vi "W7X2DPut.vi"(0 "SigLabel":string, 1 "SigJSONbuffer":string, 3 "values":T1(array[cluster]), 4 "sample rate":u16, 5 "sample period":dbl, 6 "Unit":string, 7 "pulse_length":dbl, 8 "local storage only":bool, 17 "dimensions":i64[](array[numeric])=[1399090569999999999, -1]) -> (10 "headers parms":string, 12 "headers":string, 13 "Parlog error out":errorcluster, 14 "body":string, 15 "body Parlog":string, 18 "file path written":string)   [LabVIEW 2014]
uses:
  <vilib>/httpClient/POSTBuffer.vi
  <vilib>/httpClient/LabVIEWHTTPClient.lvlib
panel:
  out "JSON string":string
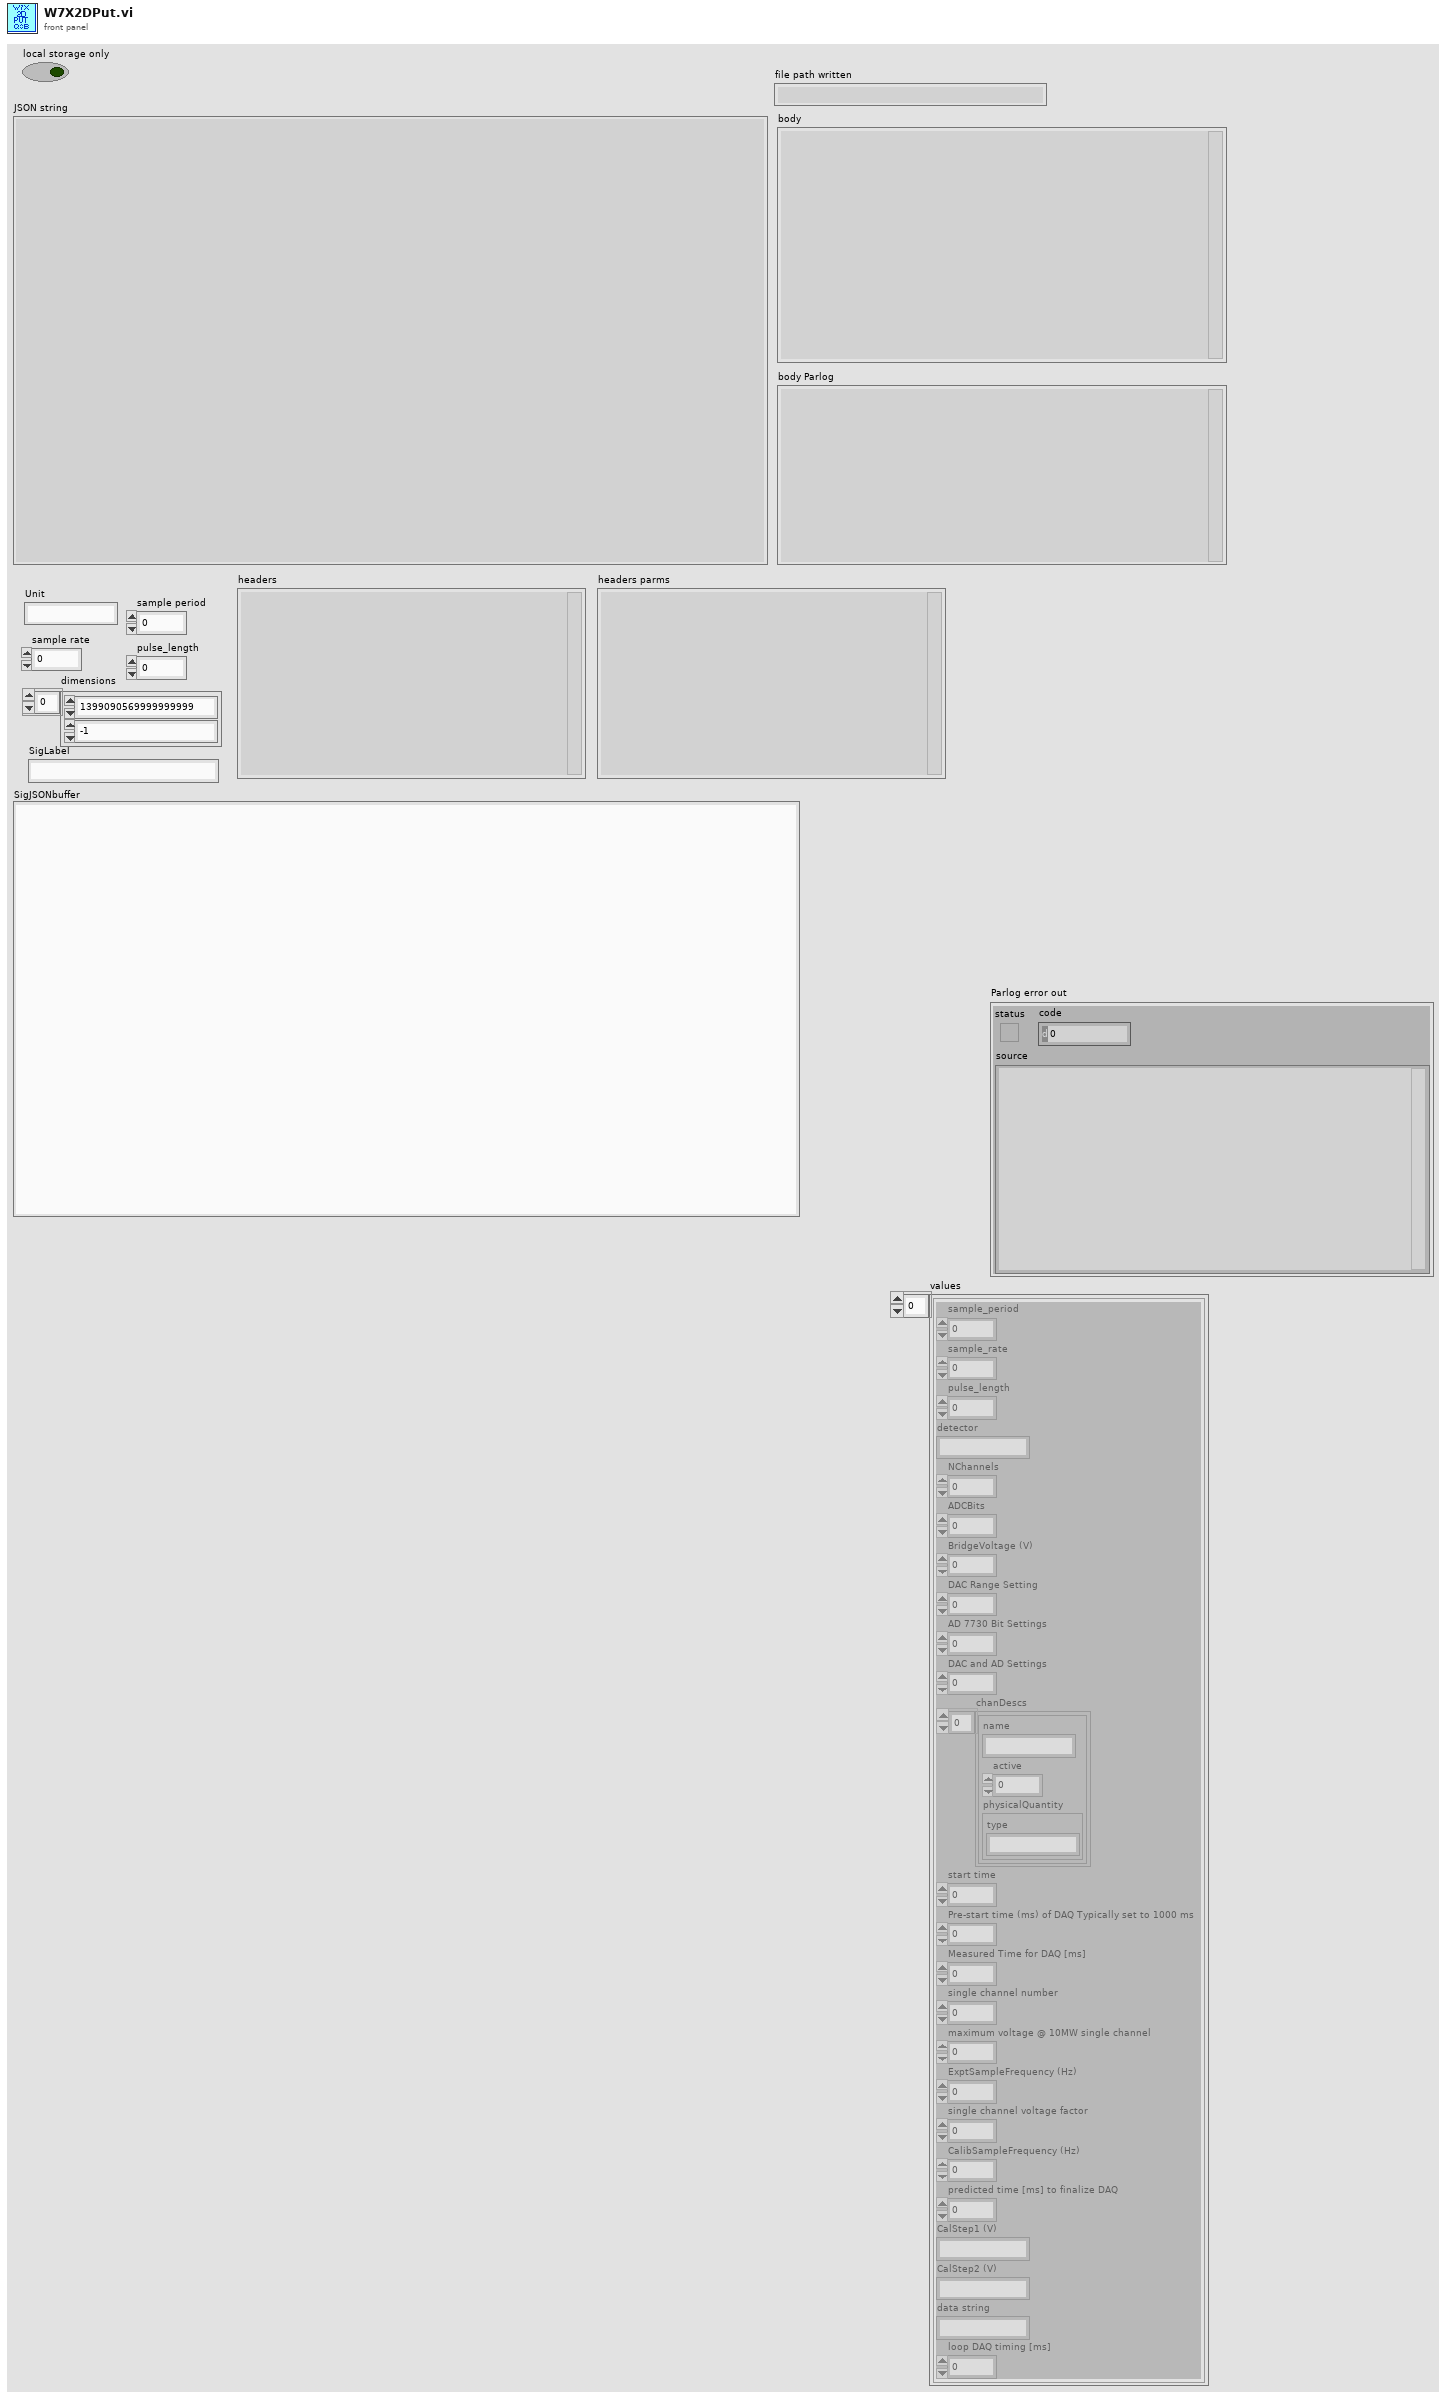
[diagram p1: front panel]
types:
  T1 = cluster{"sample_period":dbl, "sample_rate":dbl, "pulse_length":dbl, "detector":string, "NChannels":i16, "ADCBits":i16, "BridgeVoltage (V)":sgl, "DAC Range Setting":u8, "AD 7730 Bit Settings":i32, "DAC and AD Settings":i32, "chanDescs":cluster{"name":string, "active":i32, "physicalQuantity":cluster{"type":string}}[], "start time":i64, "Pre-start time (ms) of DAQ Typically set to 1000 ms":i32, "Measured Time for DAQ [ms] ":u32, "single channel number":i64, "maximum voltage @ 10MW single channel":dbl, "ExptSampleFrequency (Hz)":sgl, "single channel voltage factor":dbl, "CalibSampleFrequency (Hz)":sgl, "predicted time [ms] to finalize DAQ":dbl, "CalStep1 (V)":string, "CalStep2 (V)":string, "data string":string, "loop DAQ timing [ms]":dbl}[]
  T2 = cluster{"sample_period":dbl, "sample_rate":dbl, "pulse_length":dbl, "detector":string, "NChannels":i16, "ADCBits":i16, "BridgeVoltage (V)":sgl, "DAC Range Setting":u8, "AD 7730 Bit Settings":i32, "DAC and AD Settings":i32, "chanDescs":cluster{"name":string, "active":i32, "physicalQuantity":cluster{"type":string}}[], "start time":i64, "Pre-start time (ms) of DAQ Typically set to 1000 ms":i32, "Measured Time for DAQ [ms] ":u32, "single channel number":i64, "maximum voltage @ 10MW single channel":dbl, "ExptSampleFrequency (Hz)":sgl, "single channel voltage factor":dbl, "CalibSampleFrequency (Hz)":sgl, "predicted time [ms] to finalize DAQ":dbl, "CalStep1 (V)":string, "CalStep2 (V)":string, "data string":string, "loop DAQ timing [ms]":dbl}
  T3 = cluster{"name":string, "active":i32, "physicalQuantity":cluster{"type":string}}[]
  T4 = cluster{"name":string, "active":i32, "physicalQuantity":cluster{"type":string}}
  T5 = cluster{"label":string, "values":cluster{"sample_period":dbl, "sample_rate":dbl, "pulse_length":dbl, "detector":string, "NChannels":i16, "ADCBits":i16, "BridgeVoltage (V)":sgl, "DAC Range Setting":u8, "AD 7730 Bit Settings":i32, "DAC and AD Settings":i32, "chanDescs":cluster{"name":string, "active":i32, "physicalQuantity":cluster{"type":string}}[], "start time":i64, "Pre-start time (ms) of DAQ Typically set to 1000 ms":i32, "Measured Time for DAQ [ms] ":u32, "single channel number":i64, "maximum voltage @ 10MW single channel":dbl, "ExptSampleFrequency (Hz)":sgl, "single channel voltage factor":dbl, "CalibSampleFrequency (Hz)":sgl, "predicted time [ms] to finalize DAQ":dbl, "CalStep1 (V)":string, "CalStep2 (V)":string, "data string":string, "loop DAQ timing [ms]":dbl}[], "dimensions":i64[]}
  T6 = typedef "LabVIEWHTTPClient.lvlib/ClientHandle.ctl" = refnum<k1>
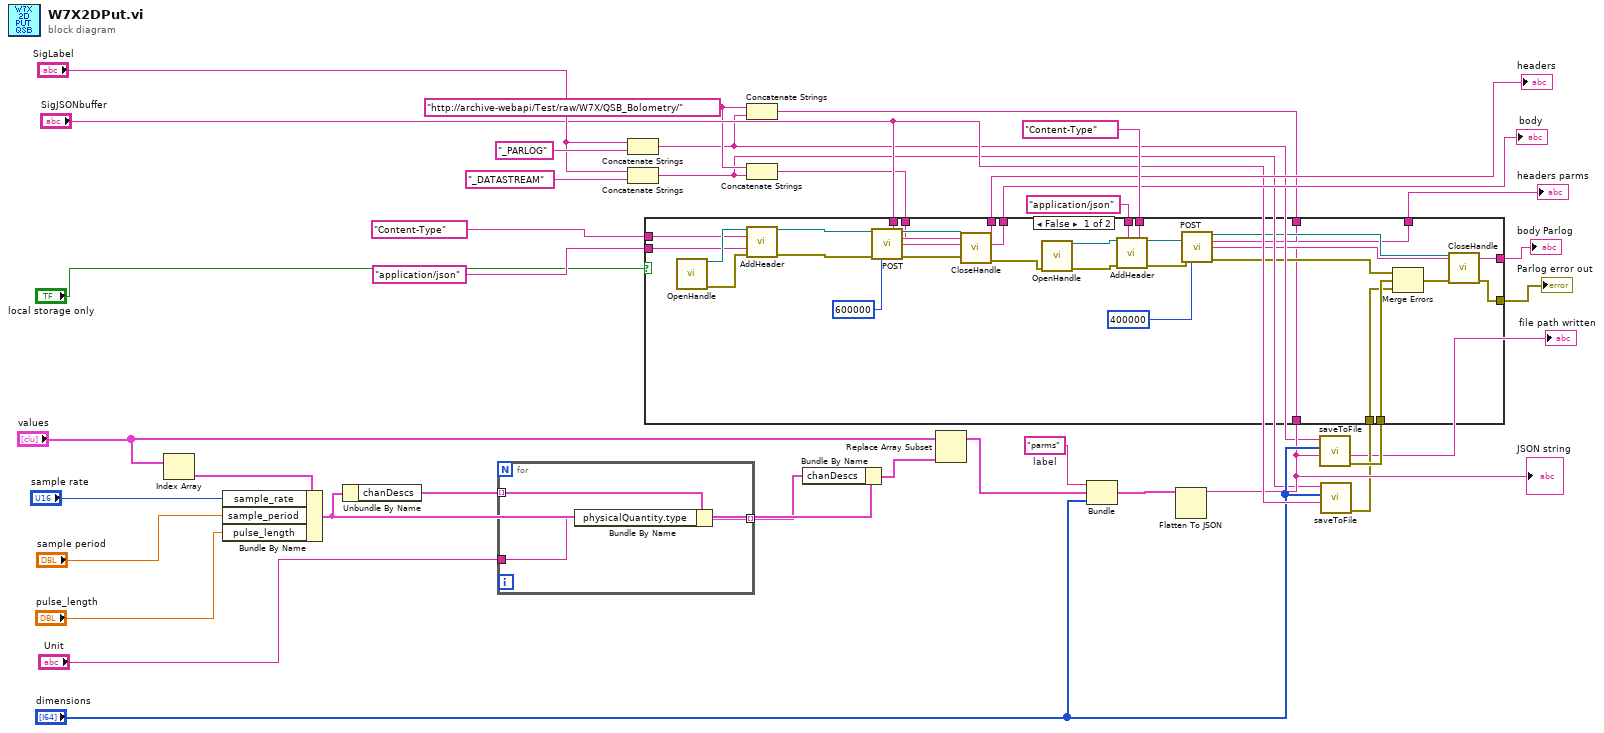
[diagram p0: block diagram]
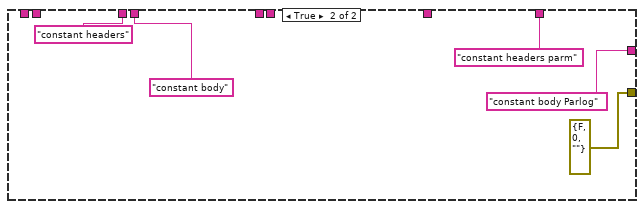
[diagram p2: hidden frame]
diagram:
  w27 = "parms"  # label
  w12 = "http://archive-webapi/Test/raw/W7X/QSB_Bolometry/" ("url")
  n1 = Index Array(array="values") -> (element=w22:T2)  [unwired: 1 in]
  n2 = Bundle By Name(cluster=w22, "sample_rate"="sample rate", "sample_period"="sample period", "pulse_length"="pulse_length") -> (w19:T2)
  n3 = Unbundle By Name(w19) -> ("chanDescs"=w18:T3)
  n4 = for {
    tunnel: w18 -> [w38] mode=indexing
    tunnel: [w40] -> w17 mode=indexing
    tunnel: "Unit" -> [w39]
    n5 = Bundle By Name(cluster=w38, "physicalQuantity.type"=w39) -> (w40:T4)
  }
  n6 = Concatenate Strings("SigLabel", "_PARLOG" ("replace string (\"\")")) -> (w7:string)
  n7 = Concatenate Strings("SigLabel", "_DATASTREAM" ("string")) -> (w6:string)
  n8 = Concatenate Strings(w12, w7) -> (w13:string)
  n9 = Concatenate Strings(w12, w6) -> (w4:string)
  n10 = Bundle By Name(cluster=w19, "chanDescs"=w17) -> (w21:T2)
  n11 = Replace Array Subset(array="values", new element=w21) -> (w20:T1)  [unwired: 1 in]
  n12 = Bundle("label"=w27, "values"=w20, "dimensions"="dimensions") -> (w26:T5)  [unwired: 1 in]
  n13 = Flatten To JSON(anything=w26) -> (JSON string=w10:string)  [unwired: 2 in, 1 out]
  "JSON string" <- w10
  n14 = call "saveToFile.vi"("SigJSONbuffer"=w10, "dimensions"="dimensions", "String"=w7) -> ("error out"=w9:errorcluster, "resulting string"=→"file path written":string)  [unwired: 7 in]
  n15 = call "saveToFile.vi"("SigJSONbuffer"="SigJSONbuffer", "dimensions"="dimensions", "String"=w6) -> ("error out"=w8:errorcluster)  [unwired: 7 in, 1 out]
  n16 = case shown="False" "local storage only" {
    tunnel: "Content-Type" ("header") -> [w65 _]
    tunnel: "application/json" ("value") -> [w64 _]
    tunnel: [w63 "constant body Parlog" ("headers")] -> w35
    tunnel: [w61 errorcluster {"status"=FALSE, "code"=0, "source"=""} ("error out")] -> w34
    tunnel: [w58 "constant headers" ("headers")] -> w33
    tunnel: "Content-Type" ("header") -> [w53 _]
    tunnel: "application/json" ("value") -> [w52 _]
    tunnel: [w51 "constant body" ("body")] -> w30
    tunnel: "SigJSONbuffer" -> [w49 _]
    tunnel: w13 -> [w48 _]
    tunnel: w10 -> [w47 _]
    tunnel: w9 -> [w45 _]
    tunnel: w8 -> [w44 _]
    tunnel: w4 -> [w42 _]
    tunnel: [w41 "constant headers parm" ("headers")] -> w3
    frame False {
      n17 = call <vilib>:"OpenHandle.vi"() -> ("client handle out"=w57:T6, "error out"=w56:errorcluster)  [unwired: 14 in]
      n18 = call <vilib>:"AddHeader.vi"("client handle"=w57, "header"=w53, "value"=w52, "error in (no error)"=w56) -> ("client handle out"=w55:T6, "error out"=w54:errorcluster)  [unwired: 10 in]
      n19 = call-poly <vilib>:"POST.vi"("client handle"=w55, "url"=w42, "buffer"=w49, "error in (no error)"=w54, "timeout (10000)"=600000) -> ("client handle out"=w60:T6, "headers"=w58:string, "body"=w51:string, "error out"=w59:errorcluster)  [unwired: 7 in]
      n20 = call <vilib>:"CloseHandle.vi"("client handle"=w60, "error in (no error)"=w59) -> ("error out"=w43:errorcluster)  [unwired: 13 in]
      n21 = call <vilib>:"OpenHandle.vi"("error in (no error)"=w43) -> ("client handle out"=w69:T6, "error out"=w68:errorcluster)  [unwired: 13 in]
      n22 = call <vilib>:"AddHeader.vi"("client handle"=w69, "header"=w65, "value"=w64, "error in (no error)"=w68) -> ("client handle out"=w67:T6, "error out"=w66:errorcluster)  [unwired: 10 in]
      n23 = call-poly <vilib>:"POST.vi"("client handle"=w67, "url"=w48, "buffer"=w47, "error in (no error)"=w66, "timeout (10000)"=400000) -> ("client handle out"=w71:T6, "headers"=w41:string, "body"=w63:string, "error out"=w70:errorcluster)  [unwired: 7 in]
      n24 = Merge Errors(w70, w45, w44) -> (w46:errorcluster)
      n25 = call <vilib>:"CloseHandle.vi"("client handle"=w71, "error in (no error)"=w46) -> ("error out"=w61:errorcluster)  [unwired: 13 in]
    }
    frame True {
    }
  }
  "Parlog error out" <- w34
  "headers parms" <- w3
  "body Parlog" <- w35
  "headers" <- w33
  "body" <- w30
